vi "m2template.vi"(8 "error in (no error)":errorcluster, 11 "class2 in":refnum<class "class2.lvclass">) -> (0 "error out":errorcluster, 3 "class2 out":refnum<class "class2.lvclass">)   [LabVIEW 2013, in "class2.lvclass"]
uses:
  class2.lvclass
  class2.lvclass/class2.ctl
panel:
  out "2D Picture ref":refnum<vi>
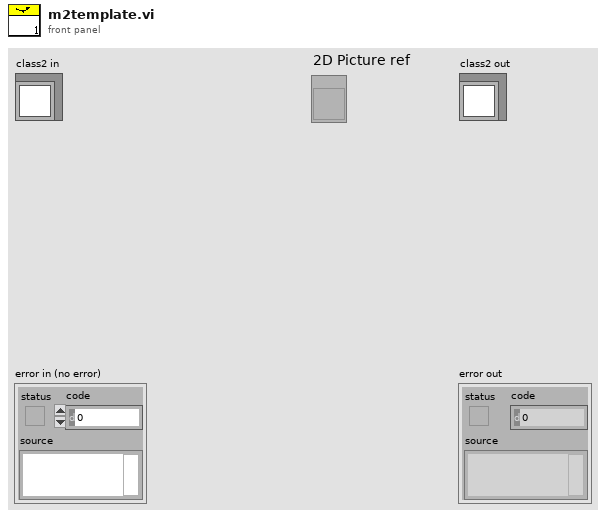
[diagram p1: front panel]
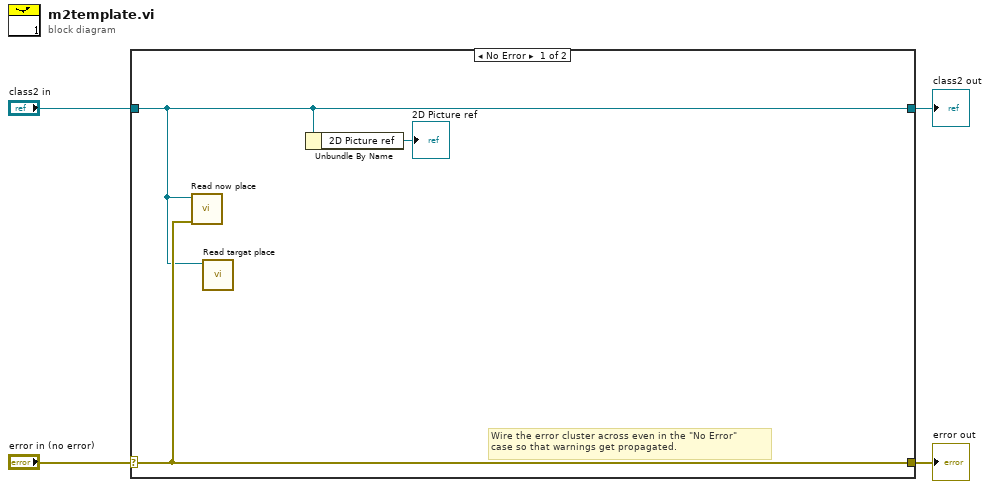
[diagram p0: block diagram]
diagram:
  n1 = case shown="No Error" "error in (no error)" {
    selector: "error in (no error)" -> [w7 w9]
    tunnel: [w7 w9] -> w3
    tunnel: [w6 w8] -> w1
    tunnel: "class2 in" -> [w6 w8]
    frame No Error {
      # "Wire the error cluster across even in the \"No Error\"\ncase so that warnings get propagated."
      n2 = call-dynamic "Read now place.vi"("error in (no error)"=w7, "mainclass in"=w6) -> ()  [unwired: 7 in, 3 out]
      n3 = call-dynamic "Read targat place.vi"("mainclass in"=w6) -> ()  [unwired: 8 in, 3 out]
      n4 = Unbundle By Name(w6) -> ("2D Picture ref"=→"2D Picture ref":refnum<vi>)
    }
    frame Error {
    }
  }
  "error out" <- w3
  "class2 out" <- w1
